vi "Write Input SGL Values.vi"(8 "error in (no error)":errorcluster, 9 "values":sgl[](array[numeric]), 10 "starting address":u16, 11 "standard data model in":refnum<class "Device Data Model.lvclass">) -> (0 "error out":errorcluster, 3 "standard data model out":refnum<class "Device Data Model.lvclass">)   [LabVIEW 2021, in "Device Data Model.lvclass"]
doc: "Writes the values of multiple input register values in series, starting at address M."
uses:
  Device Data Model.lvclass
  Device Data Model.lvclass/Device Data Model.ctl
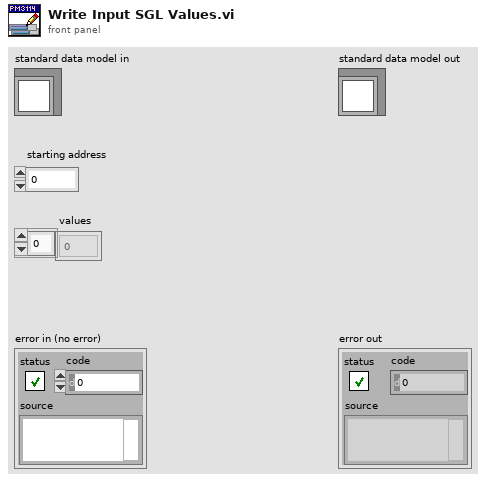
[diagram p1: front panel]
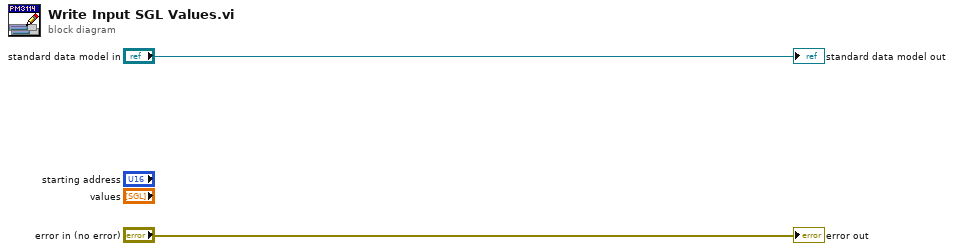
[diagram p0: block diagram]
diagram:
  "error out" <- "error in (no error)"
  "standard data model out" <- "standard data model in"
